vi "Memory.Pointer.Write.Safe.1D.SGL.vi"(8 "error in (no error)":errorcluster, 9 "count":u64 format="%d elements", 10 "buffer in":sgl[](array[numeric]), 11 "pointer in":refnum<class "Memory.Pointer.lvclass">) -> (0 "error out":errorcluster, 2 "buffer out":sgl[](array[numeric]), 3 "pointer out":refnum<class "Memory.Pointer.lvclass">)   [LabVIEW 2016, in "Memory Manager.lvlib" / "Memory.Pointer.lvclass"]
doc: "Writes <b>count</b> elements from the provided <b>buffer</b> to the address specified by <b>pointer</b>.\n\n<b>Note:</b> This VI is <b>unsafe</b>.\n\nUnsafe means that it does not evaluate the size parameter of <b>pointer</b> to ensure that is inbounds of allocated memory before peforming a memory read/write. Reading/writing more data to a pointer than it has allocated can corrupt or crash LabVIEW. Only use this VI in scenarios where the <b>pointer</b> has been validated to be allocated to a correct size before calling this VI."
uses:
  Memory.Pointer.lvclass
  Memory.Pointer.lvclass/Memory.Pointer.ctl
  Accessors/Get Address.vi
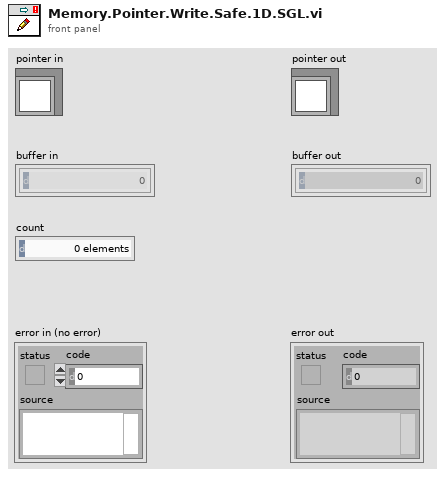
[diagram p1: front panel]
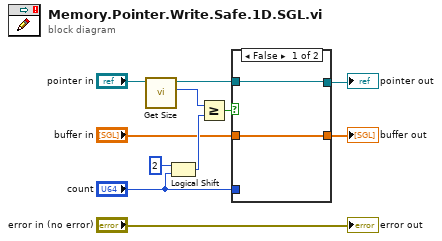
[diagram p0: block diagram]
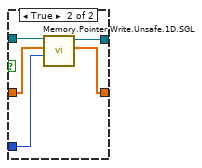
[diagram p2: hidden frame]
diagram:
  n1 = call "Get Size.vi"("Pointer in"="pointer in") -> ("size"=w7:u64, "Pointer out"=w5:refnum<class "Memory.Pointer.lvclass">)  [unwired: 8 in, 1 out]
  n2 = Logical Shift(y=i16 2, x="count") -> (x << y=w8:u64)
  n3 = Greater Or Equal?(x=w7, y=w8) -> (x >= y?=w6:bool)
  n4 = case shown="False" w6 {
    tunnel: w5 -> [w12 w18]
    tunnel: [w12 w17] -> w4
    tunnel: [w13 w16] -> w3
    tunnel: "buffer in" -> [w13 w15]
    tunnel: "count" -> [_ w14]
    frame False {
    }
    frame True {
      n5 = call "Memory.Pointer.Write.Unsafe.1D.SGL.vi"("count"=w14, "buffer in"=w15, "pointer in"=w18) -> ("buffer out"=w16:sgl[], "pointer out"=w17:refnum<class "Memory.Pointer.lvclass">)  [unwired: 6 in, 1 out]
    }
  }
  "pointer out" <- w4
  "buffer out" <- w3
  "error out" <- "error in (no error)"
